vi "PathToTemplate.vi"(10 "TemplateName":string) -> (2 "Path":path)   [LabVIEW 2017, in "MessageGen.lvlib"]
uses:
  <vilib>/addons/InsightCM/MessageBus/CodeGen/MessageGen.lvlib
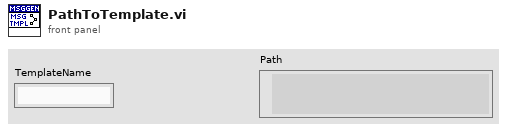
[diagram p1: front panel]
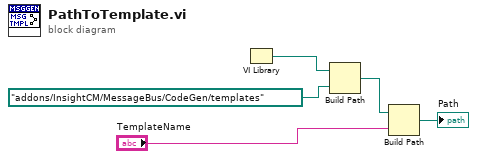
[diagram p0: block diagram]
diagram:
  n1 = VI Library() -> (path=w5:path)
  n2 = Build Path(base path=w5, name or relative path=path "addons/InsightCM/MessageBus/CodeGen/templates") -> (appended path=w3:path)
  n3 = Build Path(base path=w3, name or relative path="TemplateName") -> (appended path=→"Path":path)
